vi "SMS Image Preview Plot Data.vi"(2 "Plot Data Actions":enum16{"Read", "Write", "Reset"}(ring), 7 "Blink Number":u16) -> (8 "Plot Data":cluster{dbl[], u16[]})   [LabVIEW 2016]
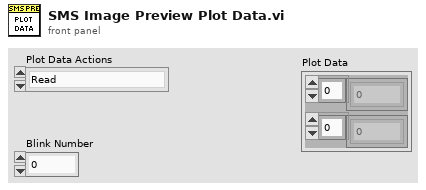
[diagram p1: front panel]
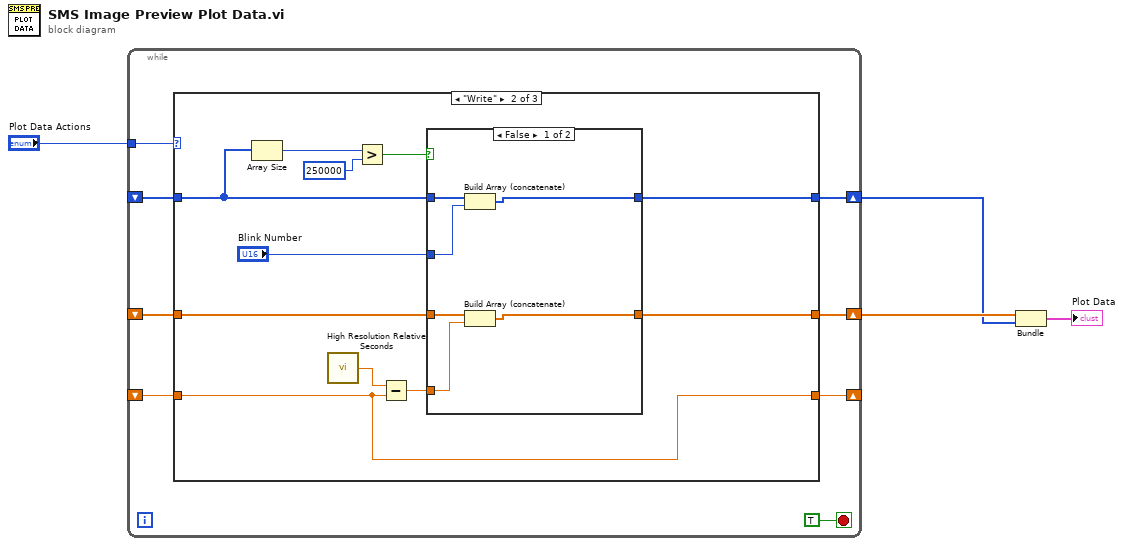
[diagram p0: block diagram]
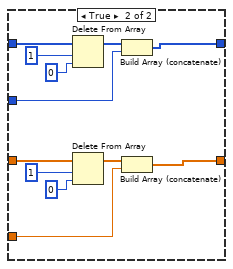
[diagram p3: hidden frame]
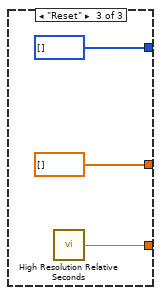
[diagram p4: hidden frame]
diagram:
  n1 = while {
    tunnel: "Plot Data Actions" -> [w11]
    shift-right: [w7] -> w2
    shift-left: _ -> [w6]
    shift-right: [w8] -> w3
    shift-left: _ -> [w5]
    shift-right: [w10] -> _
    shift-left: _ -> [w9]
    stop <- TRUE stop-if-true
    n2 = case shown="\"Write\"" w11 {
      tunnel: [w15 w16 w47] -> w10
      tunnel: w9 -> [w15 w16 _]
      tunnel: [w13 w23 dbl[] []] -> w8
      tunnel: [w14 w24 u16[] []] -> w7
      tunnel: w6 -> [w14 w21 _]
      tunnel: w5 -> [w13 w26 _]
      frame "Read", Default {
      }
      frame "Write" {
        n3 = Array Size(array=w21) -> (size(s)=w20:i32)
        n4 = call <vilib>:"High Resolution Relative Seconds.vi"() -> ("relative seconds"=w17:dbl)
        n5 = Greater?(x=w20, y=250000) -> (0:w18:bool)
        n6 = Subtract(x=w17, y=w16) -> (x-y=w22:dbl)
        n7 = case shown="False" w18 {
          tunnel: w21 -> [w32 w44]
          tunnel: w26 -> [w31 w39]
          tunnel: [w30 w36] -> w24
          tunnel: [w29 w35] -> w23
          tunnel: "Blink Number" -> [w28 w34]
          tunnel: w22 -> [w27 w33]
          frame False {
            n8 = Build Array (concatenate)(w32, w28) -> (w30:u16[])
            n9 = Build Array (concatenate)(w31, w27) -> (w29:dbl[])
          }
          frame True {
            n10 = Delete From Array(array=w44, length=1, index=0 ("length")) -> (array with subset deleted=w38:u16[])  [unwired: 1 out]
            n11 = Delete From Array(array=w39, length=1, index=0 ("length")) -> (array with subset deleted=w37:dbl[])  [unwired: 1 out]
            n12 = Build Array (concatenate)(w38, w34) -> (w36:u16[])
            n13 = Build Array (concatenate)(w37, w33) -> (w35:dbl[])
          }
        }
      }
      frame "Reset" {
        n14 = call <vilib>:"High Resolution Relative Seconds.vi"() -> ("relative seconds"=w47:dbl)
      }
    }
  }
  n15 = Bundle(w3, w2) -> (→"Plot Data":cluster{dbl[], u16[]})  [unwired: 1 in]
